vi "Shift Setting and Com Port.vi"(10 "Setting":path=path "D:/data/Test Settings") -> (2 "OK":bool)   [LabVIEW 2023]
uses:
  Controls/Communication setting.ctl
panel:
  in  "BARCODE PRINTER\nPORT":refnum<visa-resource-name>
  in  "LEAK SCANNER \nPORT":refnum<visa-resource-name>
  in  "Shift-C":timestamp format="%<%H:%M>T"
  in  "Shift-B":timestamp format="%<%H:%M>T"
  in  "Shift-A":timestamp format="%<%H:%M>T"
  in  "LIGHT SCANNER\n PORT":refnum<visa-resource-name>
  in  "OK 2":bool
  in  "Cancel":bool
  out "DATE & TIME":string="10/20/2014   5:08:59 PM"
  # "Shift Setting"
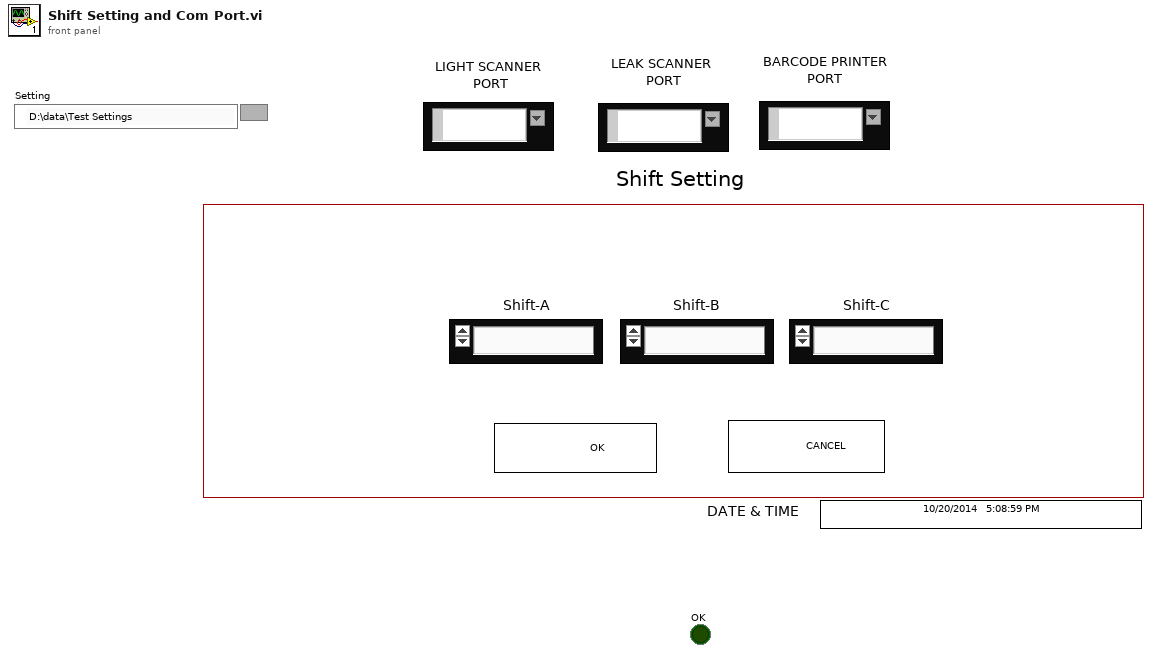
[diagram p1: front panel]
types:
  T1 = typedef "Communication setting.ctl" = cluster{"Light Scanner Port":refnum<visa-resource-name>, "Shift-A":timestamp, "Shift-B":timestamp, "Shift-C":timestamp, "Leak Scanner Port":refnum<visa-resource-name>, "Barcode Printer":refnum<visa-resource-name>}
  T2 = enum16{"open", "replace", "create", "open or create", "replace or create", "replace or create with confirmation"}
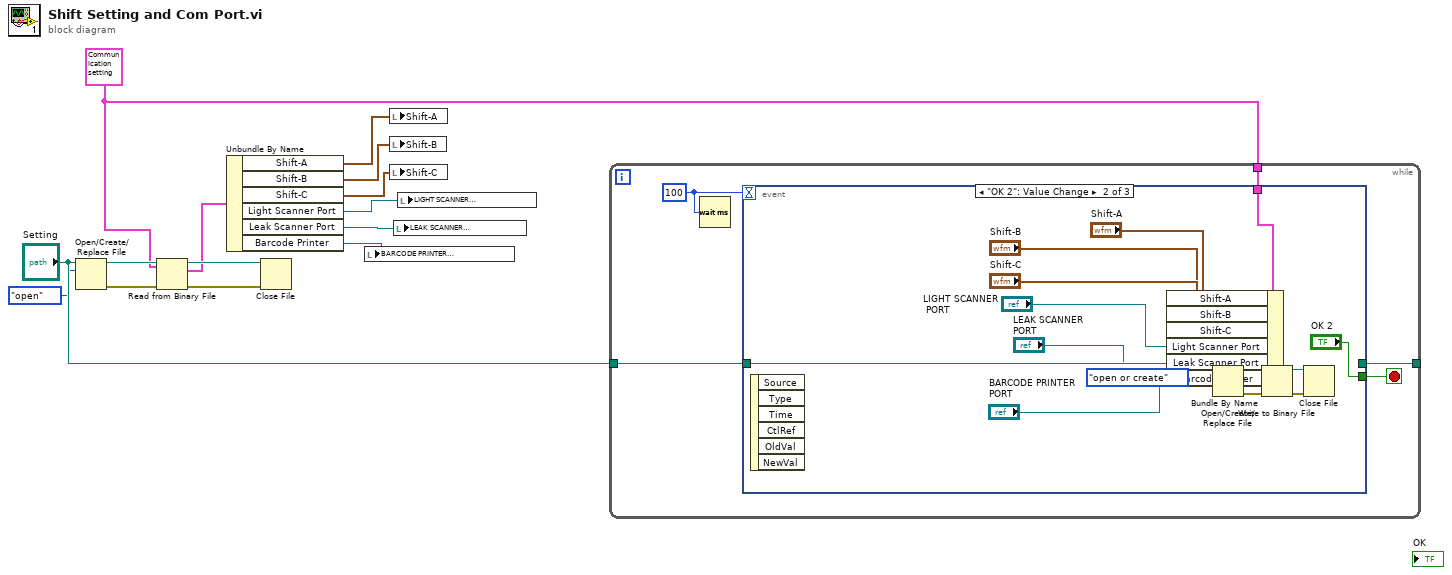
[diagram p0: block diagram]
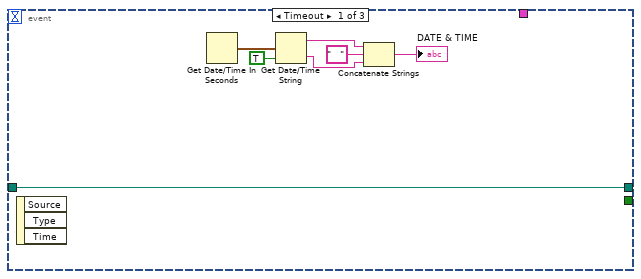
[diagram p2: hidden frame]
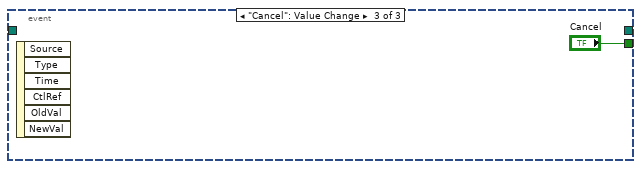
[diagram p3: hidden frame]
diagram:
  w1 = T1 {"Light Scanner Port"="", "Shift-A"=timestamp(0 s since 1904-01-01), "Shift-B"=timestamp(0 s since 1904-01-01), "Shift-C"=timestamp(0 s since 1904-01-01), "Leak Scanner Port"="", "Barcode Printer"=""} ("output cluster")
  n1 = Open/Create/Replace File(file path (use dialog)="Setting", operation (0:open)=T2."open") -> (refnum out=w12:refnum<file>, error out=w13:errorcluster)  [unwired: 4 in, 1 out]
  n2 = Read from Binary File(5:w1, 8:w13, 11:w12) -> (0:w9:errorcluster, 2:w4:T1, 3:w10:refnum<file>)  [unwired: 3 in, 1 out]
  n3 = Unbundle By Name(w4) -> ("Shift-A"=w7:timestamp, "Shift-B"=w6:timestamp, "Shift-C"=w5:timestamp, "Light Scanner Port"=w8:refnum<visa-resource-name>, "Leak Scanner Port"=w3:refnum<visa-resource-name>, "Barcode Printer"=w2:refnum<visa-resource-name>)
  n4 = Close File(refnum=w10, error in=w9) -> ()  [unwired: 2 out]
  n5 = local write "BARCODE PRINTER\nPORT"(w2) -> ()
  n6 = local write "Shift-A"(w7) -> ()
  n7 = local write "Shift-B"(w6) -> ()
  n8 = local write "Shift-C"(w5) -> ()
  n9 = local write "LEAK SCANNER \nPORT"(w3) -> ()
  n10 = local write "LIGHT SCANNER\n PORT"(w8) -> ()
  n11 = while {
    tunnel: "Setting" -> [w18]
    tunnel: [w17] -> _
    tunnel: w1 -> [w15]
    stop <- w16 stop-if-true
    w19 = u32 100 ("milliseconds to wait")
    n12 = Wait (ms)(milliseconds to wait=w19) -> ()  [unwired: 1 out]
    n13 = event shown="[1] \"OK 2\": Value Change" {
      selector: _ -> [_ _ _]
      dyn-events: _ -> [_ _ _]
      timeout: w19 -> [_ _ _]
      tunnel: w18 -> [w20 w30 _]
      tunnel: [w20 _ _] -> w17
      tunnel: [_ "OK 2" "Cancel"] -> w16
      tunnel: w15 -> [_ w28 _]
      event Timeout {
        n14 = event-data() -> ()  [unwired: 1 in, 3 out]
        n15 = Get Date/Time In Seconds() -> (seconds since 1Jan1904=w25:timestamp)
        n16 = Get Date/Time String(seconds (now)=w25, want seconds? (F)=TRUE) -> (date string=w22:string, time string=w24:string)  [unwired: 1 in]
        n17 = Concatenate Strings(w22, "   " ("string"), w24) -> (→"DATE & TIME":string)
      }
      event "OK 2": Value Change {
        n18 = event-data() -> ()  [unwired: 1 in, 6 out]
        n19 = Bundle By Name(cluster=w28, "Shift-A"="Shift-A", "Shift-B"="Shift-B", "Shift-C"="Shift-C", "Light Scanner Port"="LIGHT SCANNER\n PORT", "Leak Scanner Port"="LEAK SCANNER \nPORT", "Barcode Printer"="BARCODE PRINTER\nPORT") -> (w31:T1)
        n20 = Open/Create/Replace File(file path (use dialog)=w30, operation (0:open)=T2."open or create") -> (refnum out=w33:refnum<file>, error out=w34:errorcluster)  [unwired: 4 in, 1 out]
        n21 = Write to Binary File(file (use dialog)=w33, data=w31, error in=w34) -> (refnum out=w36:refnum<file>, error out=w35:errorcluster)  [unwired: 3 in, 1 out]
        n22 = Close File(refnum=w36, error in=w35) -> ()  [unwired: 2 out]
      }
      event "Cancel": Value Change {
        n23 = event-data() -> ()  [unwired: 1 in, 6 out]
      }
    }
  }
